vi "WaitForAnyVI_backup.vi"(8 "error in (no error)":errorcluster, 10 "Message_command In":T1={"No. of command"=14, "Parameters"=["BLM_ManualControl.vi", "BLM Position", "Within ", "10300", "10 min"], "Address"="", "Boolean"=TRUE, "No. of line"=159, "Initial Time"=timestamp(3580981392.875361 s since 1904-01-01), "Current Time"=timestamp(0 s since 1904-01-01), "Status"="Wait for VI value ", "Sequence Ref."=refnum, "Temp check"=0, "Sequence_History"="Set Parameter BLM_ManualControl.vi, New position, 10300, Number\rSet Parameter BLM_ManualControl.vi, Run, 1, Boolean\r", "Subsequence"=[]}, 11 "Command Queue In":T2) -> (0 "error out":errorcluster, 2 "Message_command Out":T1={"No. of command"=14, "Parameters"=["BLM_ManualControl.vi", "BLM Position", "Within ", "10300", "10 min"], "Address"="", "Boolean"=TRUE, "No. of line"=159, "Initial Time"=timestamp(3580981392.875361 s since 1904-01-01), "Current Time"=timestamp(0 s since 1904-01-01), "Status"="Wait for BLM_ManualControl.vi BLM Position value 0.0000  Within  10300 \nTime out: 10 min \nElapsed Time: 600.1013 sec", "Sequence Ref."=refnum, "Temp check"=0, "Sequence_History"="Set Parameter BLM_ManualControl.vi, New position, 10300, Number\rSet Parameter BLM_ManualControl.vi, Run, 1, Boolean\r", "Subsequence"=[]}, 3 "Command Queue out":T2)   [LabVIEW 2020]
uses:
  Command_Queue.ctl
  Command_Message.ctl
panel:
  in  "send timeout error?":bool=TRUE
  in  "in range window":dbl=0.01
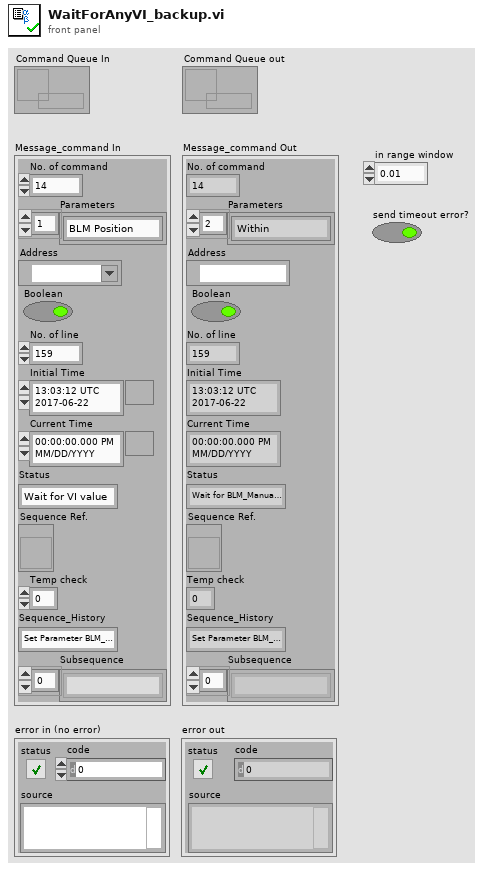
[diagram p1: front panel]
types:
  T1 = typedef "Command_Message.ctl" = cluster{"No. of command":i32, "Parameters":string[], "Address":refnum<visa-resource-name>, "Boolean":bool, "No. of line":i32, "Initial Time":timestamp, "Current Time":timestamp, "Status":string, "Sequence Ref.":refnum<vi>, "Temp check":i32, "Sequence_History":string, "Subsequence":string[]}
  T2 = typedef "Command_Queue.ctl" = refnum<queue>
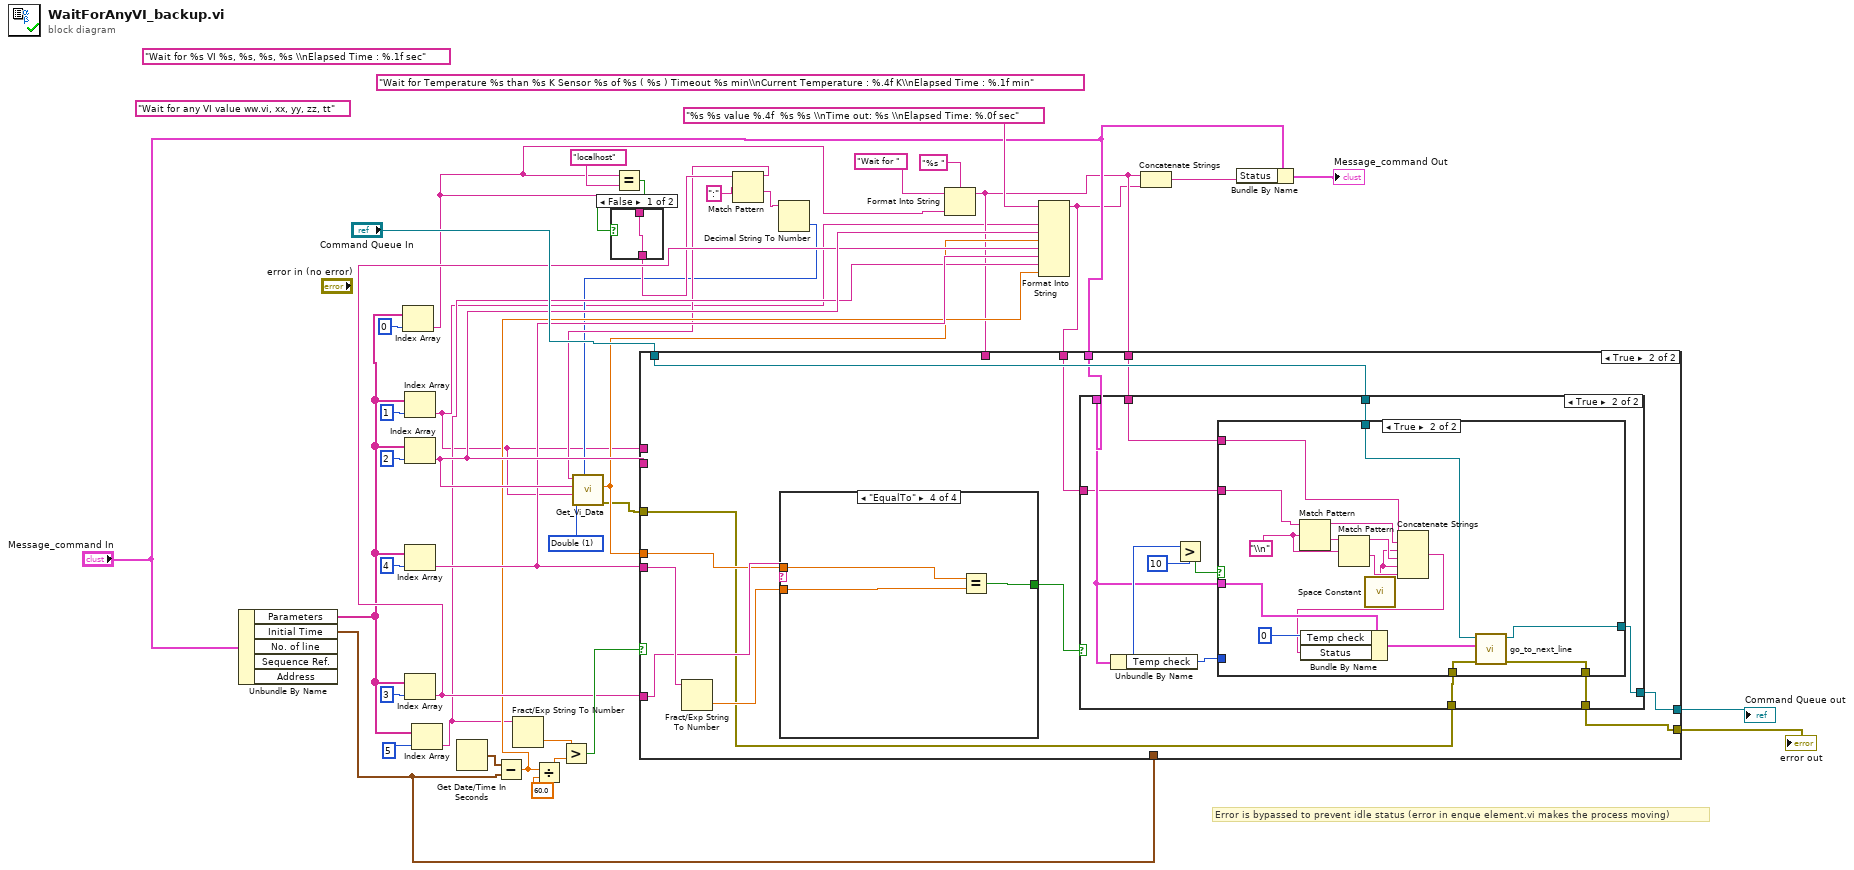
[diagram p0: block diagram]
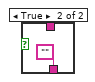
[diagram p2: hidden frame]
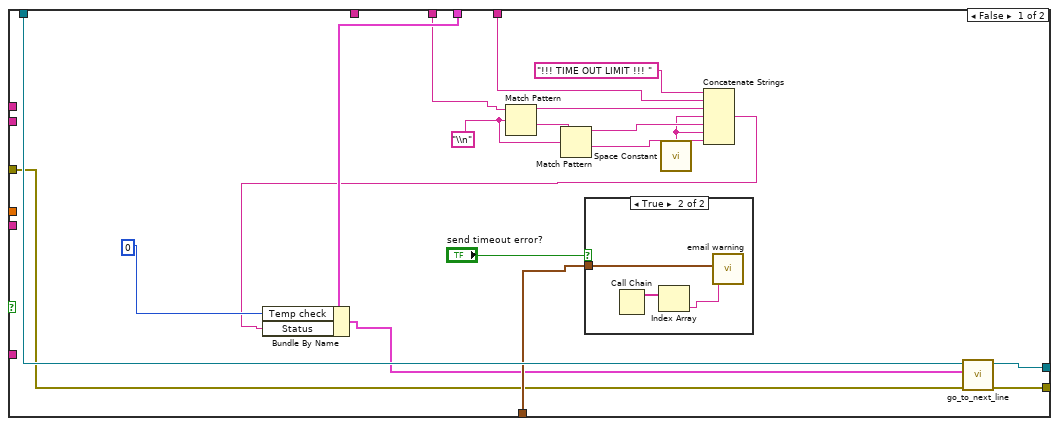
[diagram p3: hidden frame]
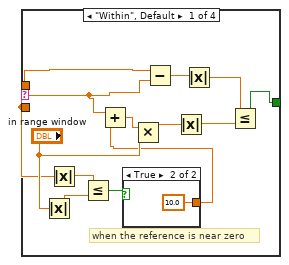
[diagram p5: hidden frame]
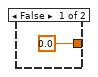
[diagram p6: hidden frame]
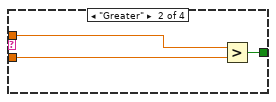
[diagram p7: hidden frame]
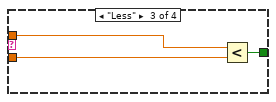
[diagram p8: hidden frame]
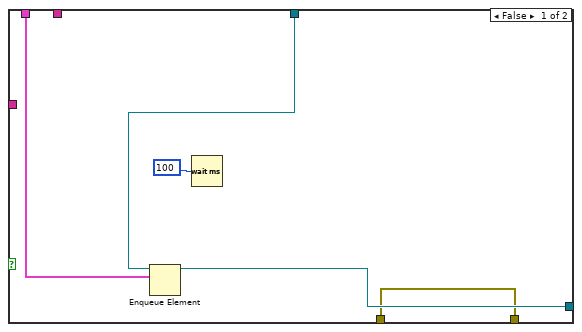
[diagram p9: hidden frame]
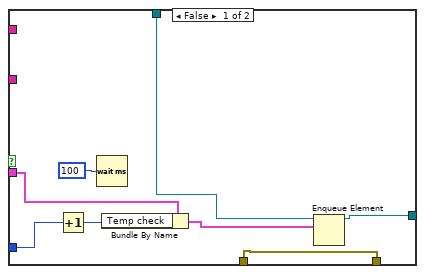
[diagram p10: hidden frame]
diagram:
  w9 = u16 1 items=["String", "Double", "Boolean", "Variant"] ("Data Type")
  (unwired) "Wait for Temperature %s than %s K Sensor %s of %s ( %s ) Timeout %s min\\nCurrent Temperature : %.4f K\\nElapsed Time : %.1f min"
  (unwired) "Wait for any VI value ww.vi, xx, yy, zz, tt" ("format string")
  (unwired) "Wait for %s VI %s, %s, %s, %s \\nElapsed Time : %.1f sec" ("format string")
  # "Error is bypassed to prevent idle status (error in enque element.vi makes the process moving)"
  n1 = Unbundle By Name("Message_command In") -> ("Parameters"=w21:string[], "Initial Time"=w23:timestamp)  [unwired: 3 out]
  n2 = Index Array(array=w21, index=0) -> (element=w10:string)
  n3 = Index Array(array=w21, index=1) -> (element=w1:string)
  n4 = Index Array(array=w21, index=2) -> (element=w28:string)
  n5 = Index Array(array=w21, index=4) -> (element=w27:string)
  n6 = Index Array(array=w21, index=3) -> (element=w26:string)
  n7 = Index Array(array=w21, index=5) -> (element=w24:string)
  n8 = Get Date/Time In Seconds() -> (seconds since 1Jan1904=w35:timestamp)
  n9 = Subtract(x=w35, y=w23) -> (x-y=w25:dbl)
  n10 = Fract/Exp String To Number(string=w24) -> (number=w34:dbl)  [unwired: 3 in, 1 out]
  n11 = Divide(x=w25, y=60.0) -> (x/y=w33:dbl)
  n12 = Greater?(x=w34, y=w33) -> (0:w32:bool)
  n13 = Equal?(x=w10, y="localhost") -> (x = y?=w14:bool)
  n14 = case shown="False" w14 {
    tunnel: [w42 ""] -> w13
    tunnel: w10 -> [w42 _]
    frame False {
    }
    frame True {
    }
  }
  n15 = Match Pattern(string=w13, regular expression=":") -> (before substring=w12:string, after substring=w16:string)  [unwired: 1 in, 2 out]
  n16 = Decimal String To Number(string=w16) -> (number=w11:i32)  [unwired: 2 in, 1 out]
  n17 = call "Get_Vi_Data.vi"("port number"=w11, "Data Type"=w9, "VI name"=w1, "Control Name"=w28, "Data mac ip address"=w12) -> ("error out"=w3:errorcluster, "Data (Double)"=w8:dbl)  [unwired: 2 in, 3 out]
  n18 = Format Into String(format string="%s ", initial string="Wait for " ("format string"), w10) -> (resulting string=w5:string)  [unwired: 1 in, 1 out]
  n19 = Format Into String(format string="%s %s value %.4f  %s %s \\nTime out: %s \\nElapsed Time: %.0f sec", w1, w28, w8, w26, w27, w24, w25) -> (resulting string=w4:string)  [unwired: 2 in, 1 out]
  n20 = case shown="True" w32 {
    tunnel: w1 -> [_ _]
    tunnel: w28 -> [_ _]
    tunnel: w27 -> [_ w77]
    tunnel: w26 -> [_ w72]
    tunnel: "Message_command In" -> [w59 w70]
    tunnel: "Command Queue In" -> [w61 w76]
    tunnel: [w60 w75] -> w30
    tunnel: w23 -> [w58 _]
    tunnel: w8 -> [_ w71]
    tunnel: w5 -> [_ _]
    tunnel: w5 -> [w53 w69]
    tunnel: w4 -> [w52 w68]
    tunnel: w3 -> [w45 w67]
    tunnel: [w44 w66] -> w2
    frame False {
      w56 = "\\n"
      n21 = Match Pattern(string=w52, regular expression=w56) -> (before substring=w55:string, after substring=w54:string)  [unwired: 1 in, 2 out]
      n22 = Match Pattern(string=w54, regular expression=w56) -> (before substring=w47:string, after substring=w48:string)  [unwired: 1 in, 2 out]
      n23 = case shown="True" "send timeout error?" {
        tunnel: w58 -> [_ w65]
        frame False {
        }
        frame True {
          n24 = Call Chain() -> (call chain=w64:string[])
          n25 = Index Array(array=w64) -> (element=w63:string)  [unwired: 1 in]
          n26 = call "email warning.vi"("running VI"=w63, "Initial"=w65) -> ()  [unwired: 9 in, 1 out]
        }
      }
      n27 = call <vilib>:"Space Constant.vi"() -> ("String"=w46:string)
      n28 = Concatenate Strings("!!! TIME OUT LIMIT !!! " ("string"), w53, w55, w46, w47, w46, w48) -> (w50:string)
      n29 = Bundle By Name(cluster=w59, "Temp check"=0, "Status"=w50) -> (w49:T1)
      n30 = call "go_to_next_line.vi"("error in (no error)"=w45, "Message_command in"=w49, "Command Queue in"=w61) -> ("error out"=w44:errorcluster, "Command Queue out"=w60:T2)  [unwired: 7 in]
    }
    frame True {
      n31 = Fract/Exp String To Number(string=w77) -> (number=w74:dbl)  [unwired: 3 in, 1 out]
      n32 = case shown="\"EqualTo\"" w72 {
        tunnel: w71 -> [w82 w95 w98 w101]
        tunnel: w74 -> [w80 w94 w97 w100]
        tunnel: [w87 w93 w96 w99] -> w73
        frame "Within", Default {
          # "when the reference is near zero"
          n33 = Absolute Value(x="in range window") -> (abs(x)=w83:dbl)
          n34 = Absolute Value(x=w80) -> (abs(x)=w84:dbl)
          n35 = Less Or Equal?(x=w84, y=w83) -> (x <= y?=w85:bool)
          n36 = case shown="True" w85 {
            tunnel: [0.0 ("in range window") 10.0 ("in range window")] -> w79
            frame False {
            }
            frame True {
            }
          }
          n37 = Add(x=w80, y=w79) -> (x+y=w81:dbl)
          n38 = Multiply(x=w81, y="in range window") -> (x*y=w89:dbl)
          n39 = Subtract(x=w82, y=w80) -> (x-y=w90:dbl)
          n40 = Absolute Value(x=w89) -> (abs(x)=w88:dbl)
          n41 = Absolute Value(x=w90) -> (abs(x)=w78:dbl)
          n42 = Less Or Equal?(x=w78, y=w88) -> (x <= y?=w87:bool)
        }
        frame "Greater" {
          n43 = Greater?(x=w95, y=w94) -> (0:w93:bool)
        }
        frame "Less" {
          n44 = Less?(x=w98, y=w97) -> (x < y?=w96:bool)
        }
        frame "EqualTo" {
          n45 = Equal?(x=w101, y=w100) -> (x = y?=w99:bool)
        }
      }
      n46 = case shown="True" w73 {
        tunnel: w70 -> [w104 w113]
        tunnel: w76 -> [w105 w112]
        tunnel: [w103 w111] -> w75
        tunnel: w69 -> [_ w110]
        tunnel: w68 -> [_ w109]
        tunnel: w67 -> [w102 w108]
        tunnel: [w102 w107] -> w66
        frame False {
          n47 = Enqueue Element(queue=w105, element=w104) -> (queue out=w103:T2)  [unwired: 2 in, 2 out]
          n48 = Wait (ms)(milliseconds to wait=u32 100) -> ()  [unwired: 1 out]
        }
        frame True {
          n49 = Unbundle By Name(w113) -> ("Temp check"=w114:i32)
          n50 = Greater?(x=w114, y=10) -> (0:w115:bool)
          n51 = case shown="True" w115 {
            tunnel: [w123 w140] -> w111
            tunnel: w114 -> [w121 _]
            tunnel: w113 -> [w119 w138]
            tunnel: w112 -> [w118 w137]
            tunnel: w110 -> [_ w132]
            tunnel: w109 -> [_ w133]
            tunnel: w108 -> [w117 w126]
            tunnel: [w117 w125] -> w107
            frame False {
              n52 = Increment(x=w121) -> (x+1=w124:i32)
              n53 = Wait (ms)(milliseconds to wait=u32 100) -> ()  [unwired: 1 out]
              n54 = Bundle By Name(cluster=w119, "Temp check"=w124) -> (w120:T1)
              n55 = Enqueue Element(queue=w118, element=w120) -> (queue out=w123:T2)  [unwired: 2 in, 2 out]
            }
            frame True {
              w136 = "\\n"
              n56 = Match Pattern(string=w133, regular expression=w136) -> (before substring=w135:string, after substring=w134:string)  [unwired: 1 in, 2 out]
              n57 = Match Pattern(string=w134, regular expression=w136) -> (before substring=w128:string, after substring=w129:string)  [unwired: 1 in, 2 out]
              n58 = call <vilib>:"Space Constant.vi"() -> ("String"=w127:string)
              n59 = Concatenate Strings(w132, w135, w127, w128, w127, w129) -> (w131:string)
              n60 = Bundle By Name(cluster=w138, "Temp check"=0, "Status"=w131) -> (w130:T1)
              n61 = call "go_to_next_line.vi"("error in (no error)"=w126, "Message_command in"=w130, "Command Queue in"=w137) -> ("error out"=w125:errorcluster, "Command Queue out"=w140:T2)  [unwired: 7 in]
            }
          }
        }
      }
    }
  }
  "Command Queue out" <- w30
  "error out" <- w2
  n62 = Concatenate Strings(w5, w4) -> (w18:string)
  n63 = Bundle By Name(cluster="Message_command In", "Status"=w18) -> (→"Message_command Out":T1)
